vi "Contour Line_Plot Data (XY Graph).vi"(11 "Contour Line":T1) -> (3 "Contour Graph":cluster{dbl[], dbl[]}(graph))   [LabVIEW 2020, in "NI_AAL_Geometry.lvlib"]
uses:
  <vilib>/Analysis/NI_AAL_Geometry.lvlib
  <vilib>/Analysis/geometry.llb/Contour Lines Control.ctl
  <vilib>/Analysis/geometry.llb/Contour Line Segment.ctl
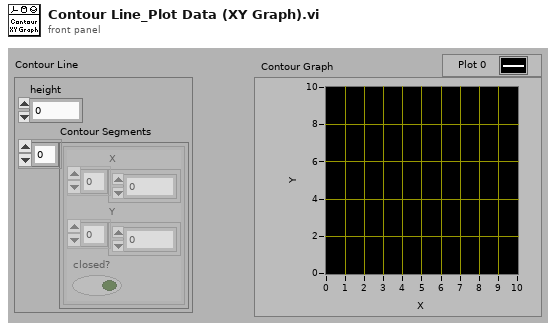
[diagram p1: front panel]
types:
  T1 = typedef "NI_AAL_Geometry.lvlib/Contour Lines Control.ctl" = cluster{"height":dbl, "Contour Segments":T2[]}
  T2 = typedef "NI_AAL_Geometry.lvlib/Contour Line Segment.ctl" = cluster{"X":dbl[], "Y":dbl[], "closed?":bool}
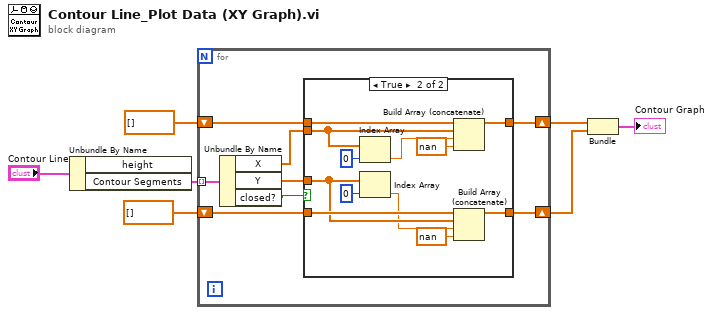
[diagram p0: block diagram]
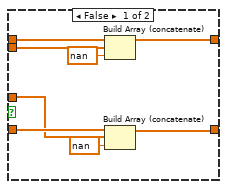
[diagram p2: hidden frame]
diagram:
  n1 = Unbundle By Name("Contour Line") -> ("Contour Segments"=w7:T2[])  [unwired: 1 out]
  n2 = for {
    tunnel: w7 -> [w15] mode=indexing
    shift-right: [w11] -> w4
    shift-left: dbl[] [] -> [w13]
    shift-right: [w9] -> w3
    shift-left: dbl[] [] -> [w10]
    n3 = Unbundle By Name(w15) -> ("X"=w14:dbl[], "Y"=w12:dbl[], "closed?"=w8:bool)
    n4 = case shown="True" w8 {
      tunnel: w14 -> [w20 w29]
      tunnel: w13 -> [w22 w35]
      tunnel: w12 -> [w18 w26]
      tunnel: [w17 w34] -> w11
      tunnel: w10 -> [w19 w33]
      tunnel: [w16 w32] -> w9
      frame False {
        n5 = Build Array (concatenate)(w22, w20, nan) -> (w17:dbl[])
        n6 = Build Array (concatenate)(w19, w18, nan) -> (w16:dbl[])
      }
      frame True {
        n7 = Index Array(array=w29, index=0) -> (element=w27:dbl)
        n8 = Index Array(array=w26, index=0) -> (element=w24:dbl)
        n9 = Build Array (concatenate)(w35, w29, w27, nan) -> (w34:dbl[])
        n10 = Build Array (concatenate)(w33, w26, w24, nan) -> (w32:dbl[])
      }
    }
  }
  n11 = Bundle(w4, w3) -> (→"Contour Graph":cluster{dbl[], dbl[]})  [unwired: 1 in]
